vi "Measurement Logic.vi"() -> ()   [LabVIEW 2021, in "start-up.lvlib"]
uses:
  start-up.lvlib
  <vilib>/Plug-In SDKs/Measurements/Measure Call Context/Measure Call Context.lvclass
  Measurement Configuration.ctl
  Measurement Results.ctl
  Controls/LEDStartup_Data.ctl
  <instrlib>/niDCPower/nidcpower.llb/niDCPower Source Mode.ctl
  <instrlib>/niDCPower/nidcpower.llb/niDCPower Wait For Event - Event.ctl
  <instrlib>/niDCPower/nidcpower.llb/niDCPower Output Function.ctl
  <instrlib>/niDCPower/nidcpower.llb/niDCPower Sequence Attribute Type.ctl
  <instrlib>/niDCPower/nidcpower.llb/niDCPower Get Channel Name From String.vi
  <vilib>/Utility/error.llb/Error Cluster From Error Code.vi
  <instrlib>/niDCPower/nidcpower.llb/niDCPower Create Advanced Sequence Step With Channels.vi
  <instrlib>/niDCPower/nidcpower.llb/niDCPower Configure Digital Edge Source Trigger With Channels.vi
  <instrlib>/niDCPower/nidcpower.llb/niDCPower Configure Digital Edge Measure Trigger With Channels.vi
  <vilib>/ErrorRing/Error Ring.xnode
panel:
  out "measurement results":T1={"Status"="Empty", "Source voltages"=[0.0], "Load voltages"=[0.0], "Source current"=[0.0], "Load current"=[0.0]}
  in  "measurement configuration":T2={"Source resource name"="", "DUT setup time"=0.5, "Source delay"=0.5, "Aperture time"=0.001, "LED voltage (Vo)"=3.06, "LED current (Io)"=0.06, "Cumulative forward voltage (Vf)"=2.83, "Source sense"=1009, "Source current limit"=2.0, "Source maximum power"=20.0, "Source start voltage"=2.7, "Source stop voltage"=5.5, "Source voltage sweep points"=10, "Load resource name"="", "Load sense"=1009, "Load voltage level range"=60.0, "Load voltage limit"=6.0, "Max output resistance"="", "Load current limit range"="", "DUT current limit"=0.0} {"DUT current limit" format="%.3f"; "LED current (Io)" format="%.2f"; "LED voltage (Vo)" format="%.3f"; "Load sense" items=["Local"=1008, "Remote"=1009]; "Source stop voltage" format="%.3f"; "Source start voltage" format="%.3f"; "Source current limit" format="%.3f"; "Source sense" items=["Local"=1008, "Remote"=1009]; "Aperture time" format="%.2p"; "Source delay" format="%#_6p"; "DUT setup time" format="%#_6p"}
  out "measure call context out":refnum<class "Measure Call Context.lvclass">
  in  "measure call context in":refnum<class "Measure Call Context.lvclass">
  out "error out":errorcluster
  in  "error in":errorcluster
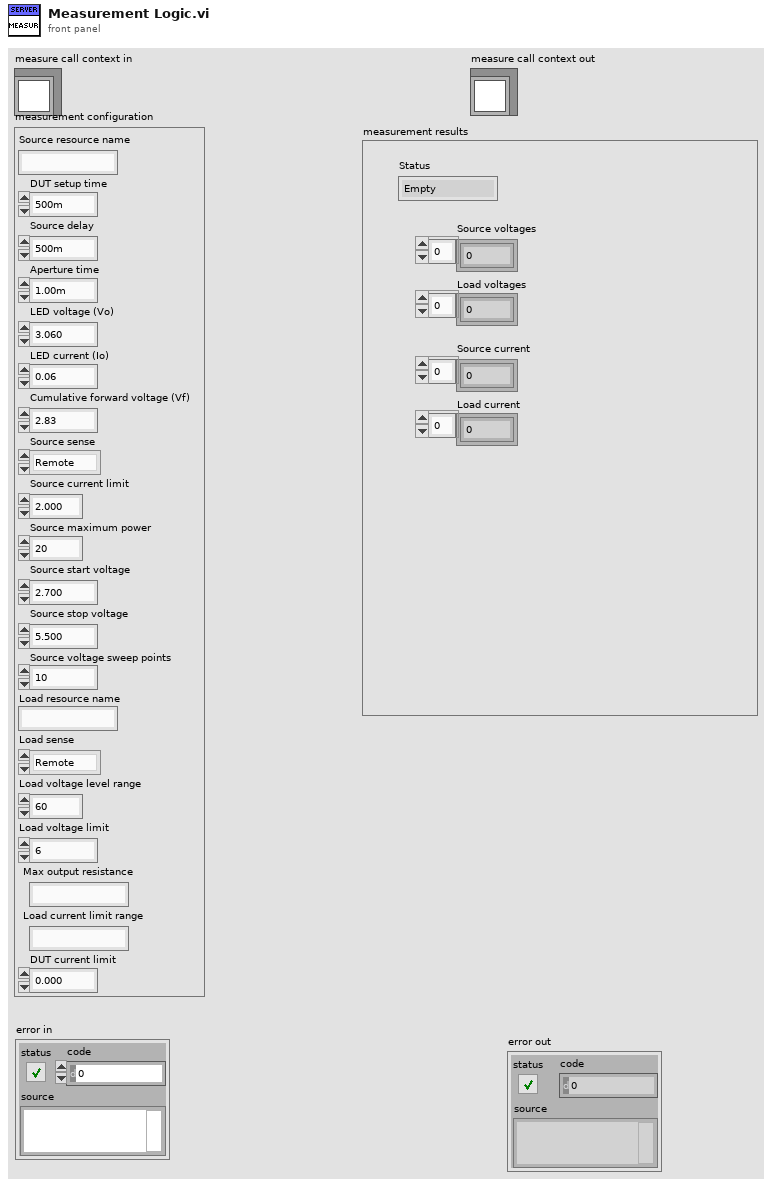
[diagram p1: front panel]
types:
  T1 = typedef "start-up.lvlib/Measurement Results.ctl" = cluster{"Status":string, "Source voltages":dbl[], "Load voltages":dbl[], "Source current":dbl[], "Load current":dbl[]}
  T2 = typedef "start-up.lvlib/Measurement Configuration.ctl" = cluster{"Source resource name":string, "DUT setup time":dbl, "Source delay":dbl, "Aperture time":dbl, "LED voltage (Vo)":dbl, "LED current (Io)":dbl, "Cumulative forward voltage (Vf)":dbl, "Source sense":i32, "Source current limit":dbl, "Source maximum power":dbl, "Source start voltage":dbl, "Source stop voltage":dbl, "Source voltage sweep points":i32, "Load resource name":string, "Load sense":i32, "Load voltage level range":dbl, "Load voltage limit":dbl, "Max output resistance":string, "Load current limit range":string, "DUT current limit":dbl}
  T3 = typedef "start-up.lvlib/LEDStartup_Data.ctl" = cluster{"Load channel name":string, "Load out":refnum<k15>, "Source out":refnum<k15>, "Source channel name":string, "Source sequence name":string, "Voltage values":dbl[], "Voltage values-CV":dbl[], "Voltage values-LED":dbl[], "Output Resistance-LED":dbl[], "Source terminal name":string, "Measure terminal name":string, "Load Voltage-out":dbl[], "Load Current - out":dbl[], "Source Voltage-out":dbl[], "Source Current - out":dbl[], "LED Mode Start?":bool, "LED Mode Completed?":bool, "CalculateRd":dbl, "Set LED Current Limit?":bool, "OutputVoltageOffset":dbl, "measurement results":T1}
  T4 = typedef "niDCPower Wait For Event - Event.ctl" = i32
  T5 = typedef "niDCPower Source Mode.ctl" = i32
  T6 = typedef "niDCPower Sequence Attribute Type.ctl" = i32
  T7 = typedef "niDCPower Output Function.ctl" = i32
  T8 = cluster{"Source Voltage":dbl[], "Source Current":dbl[], "Load Voltage":dbl[], "Load Current":dbl[]}
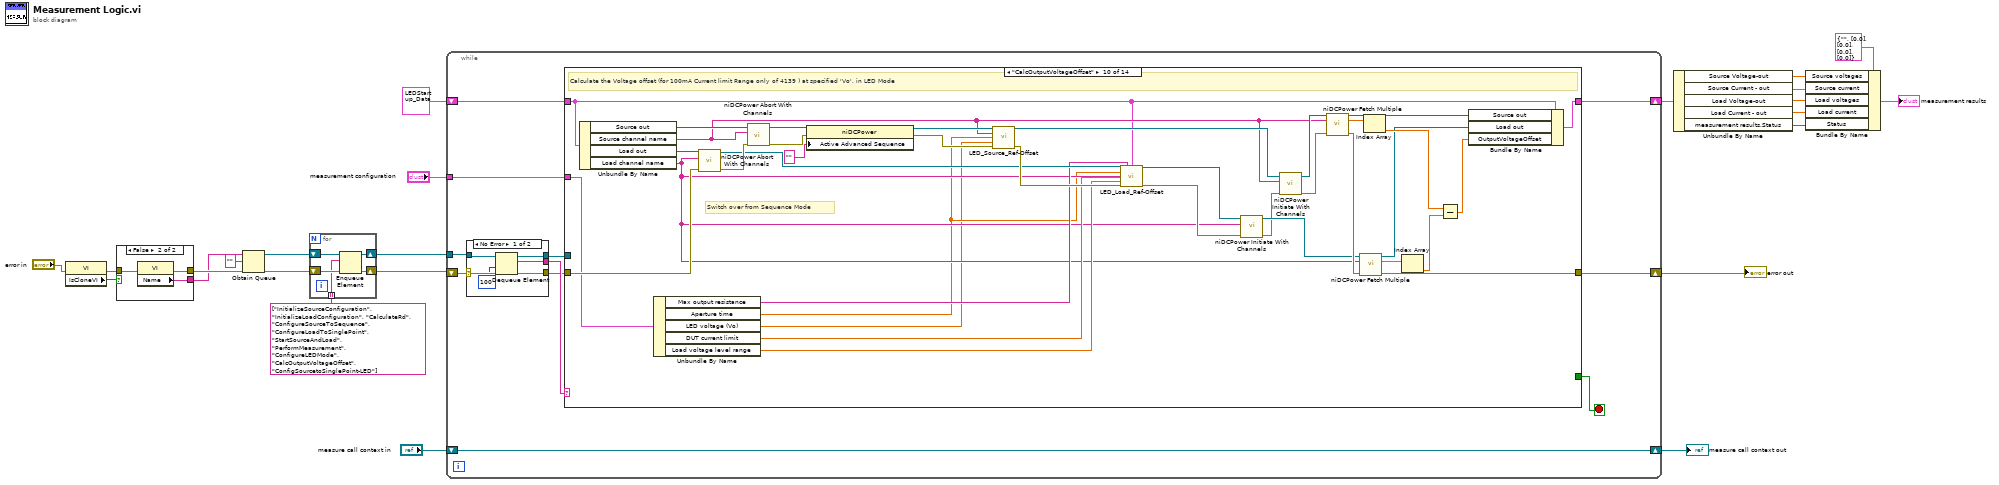
[diagram p0: block diagram]
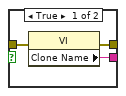
[diagram p2: hidden frame]
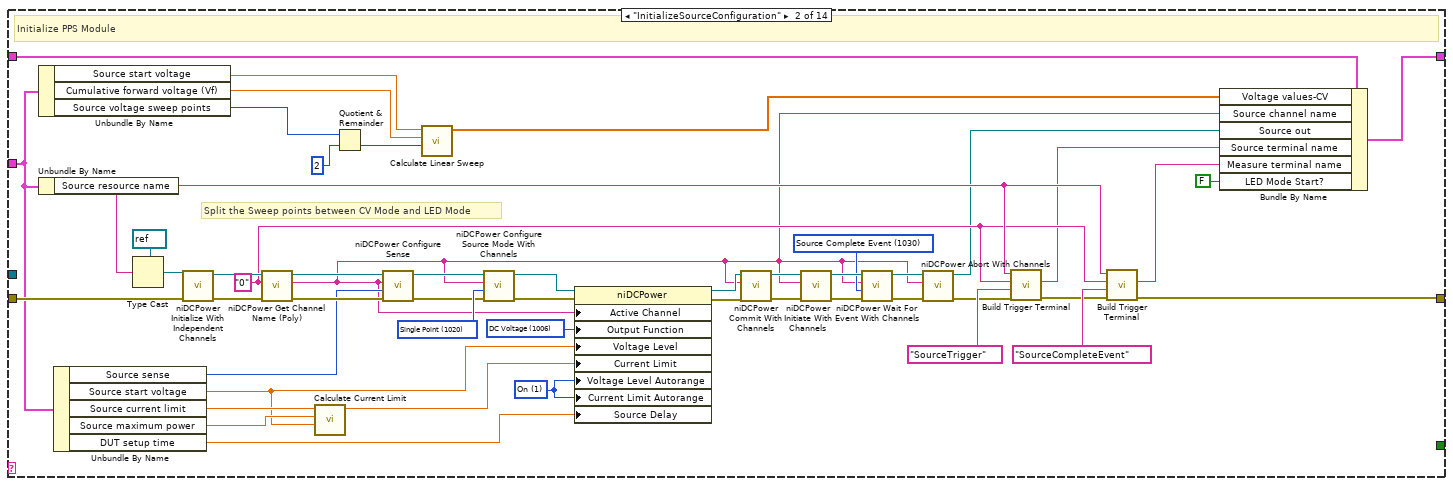
[diagram p4: hidden frame]
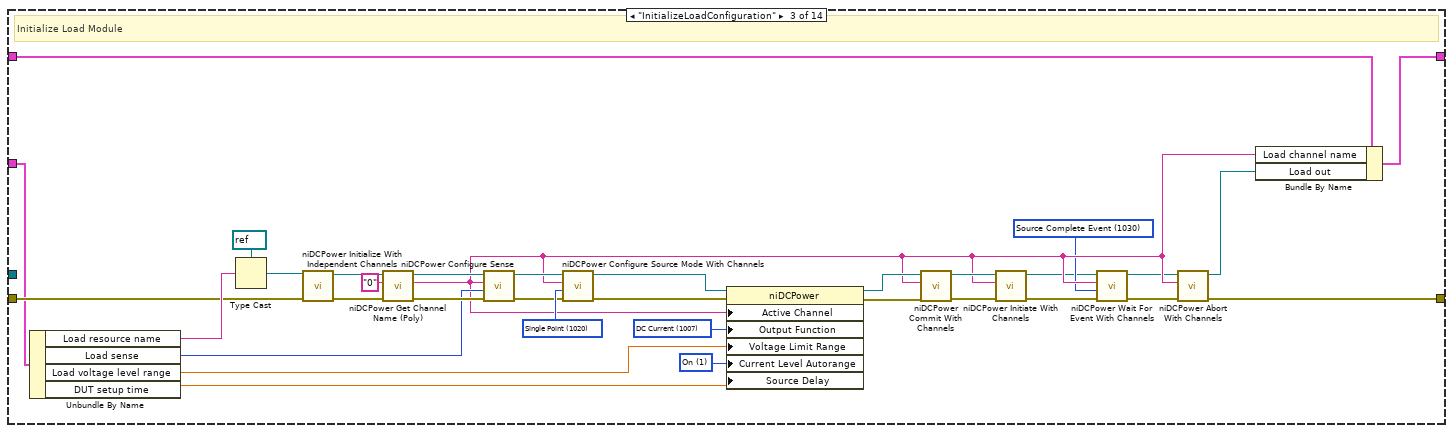
[diagram p5: hidden frame]
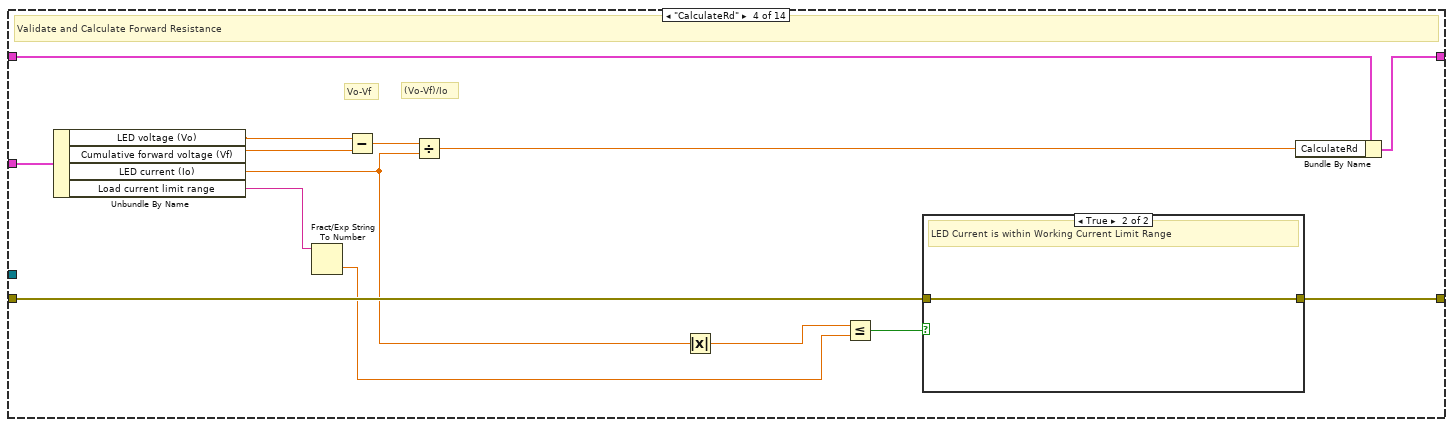
[diagram p6: hidden frame]
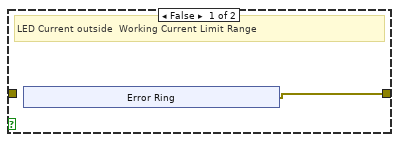
[diagram p7: hidden frame]
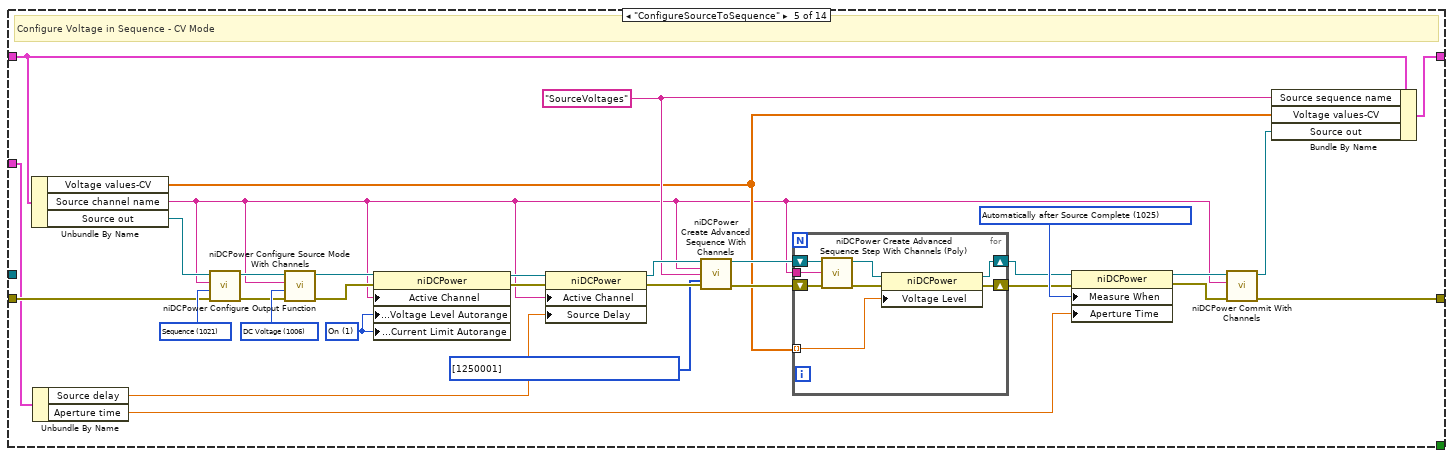
[diagram p8: hidden frame]
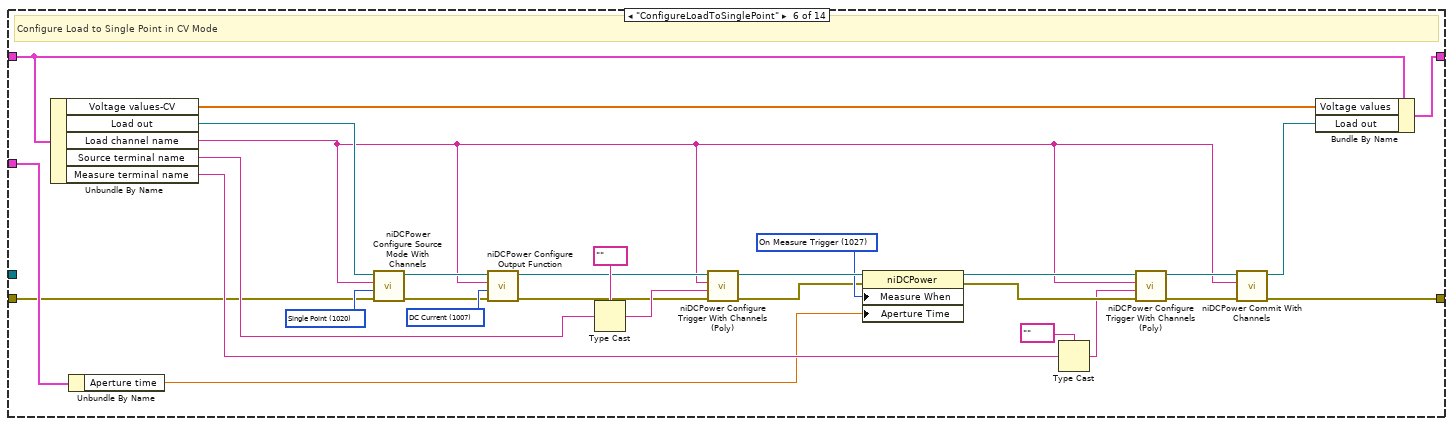
[diagram p9: hidden frame]
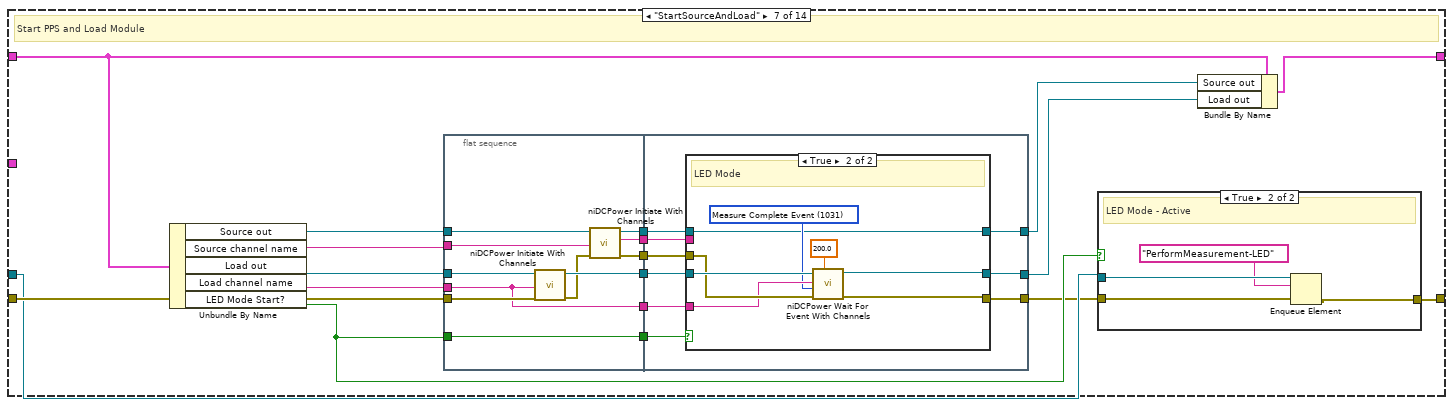
[diagram p10: hidden frame]
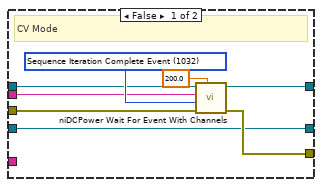
[diagram p12: hidden frame]
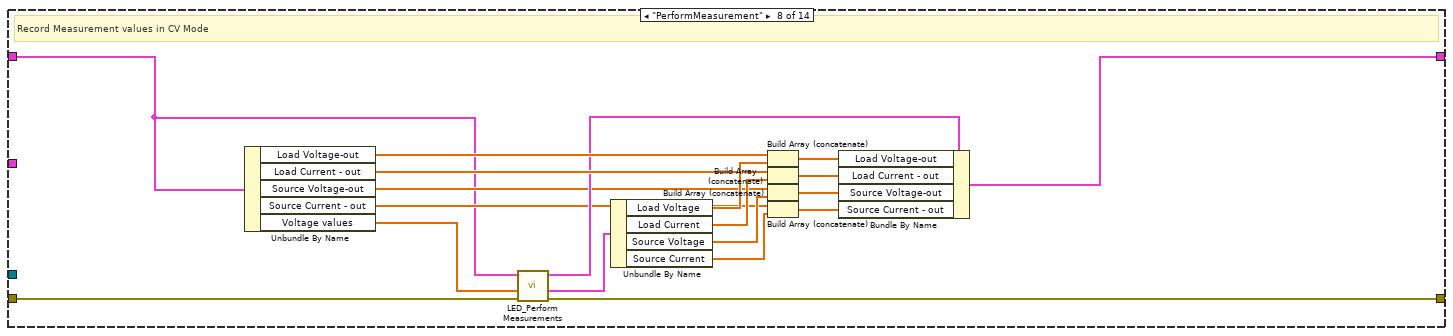
[diagram p13: hidden frame]
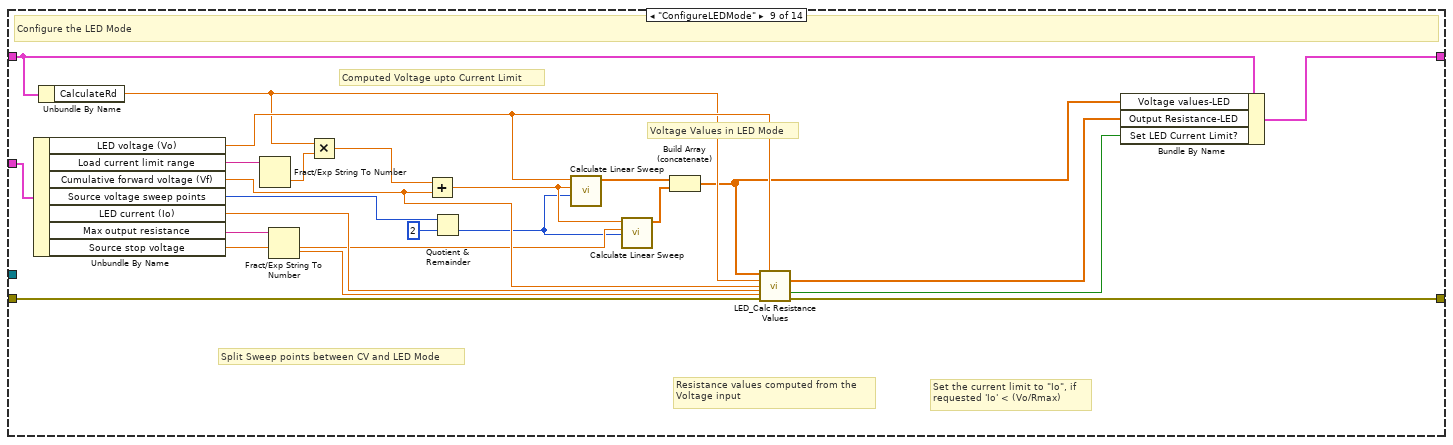
[diagram p14: hidden frame]
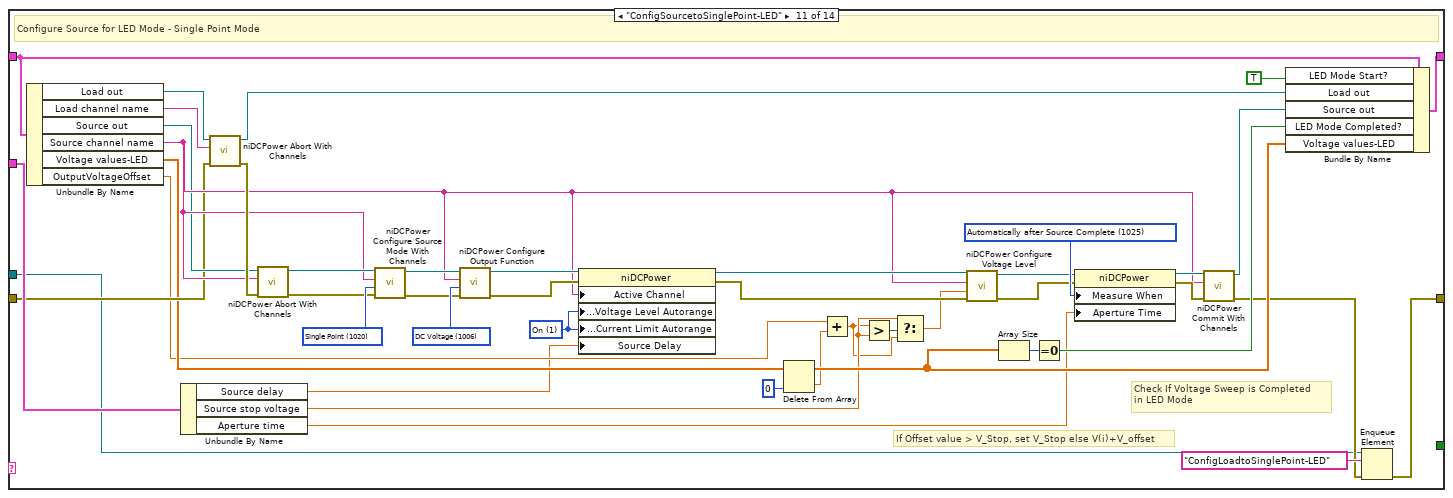
[diagram p15: hidden frame]
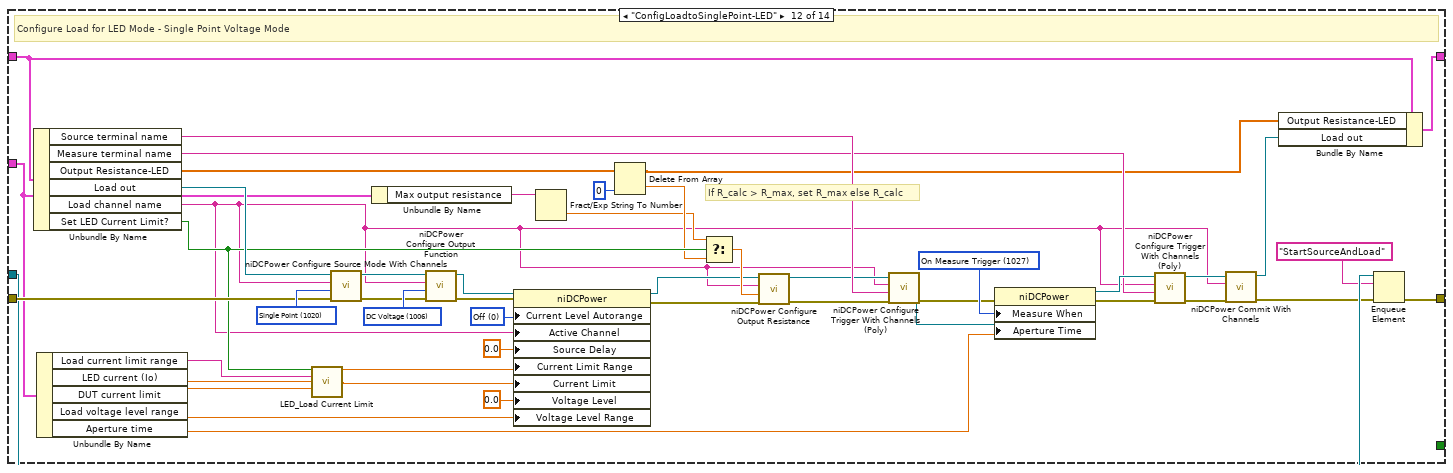
[diagram p16: hidden frame]
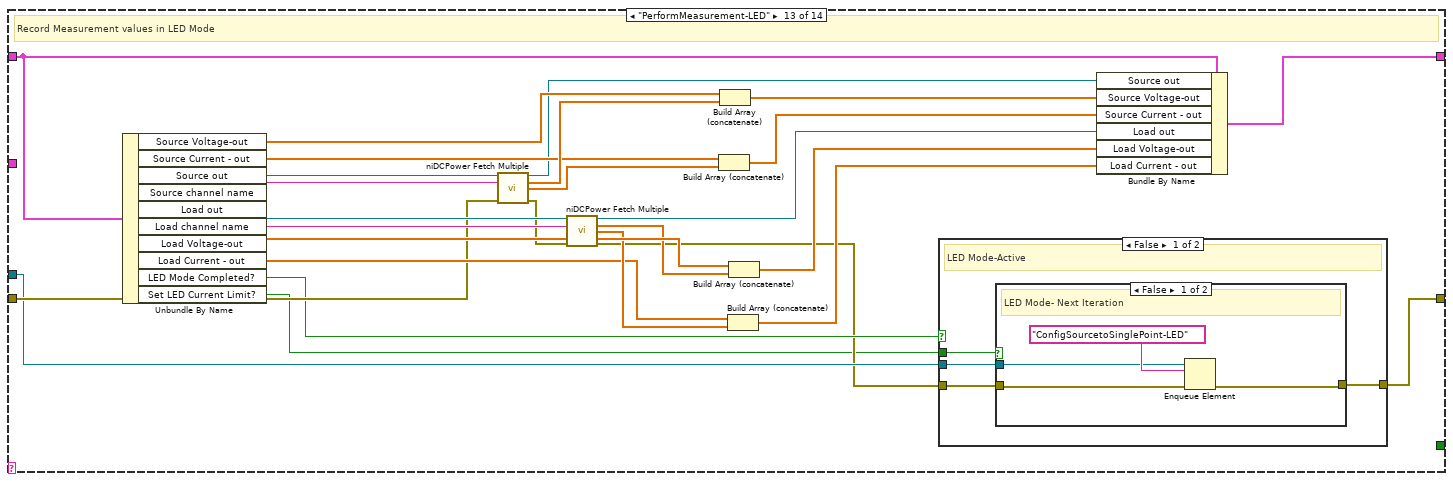
[diagram p17: hidden frame]
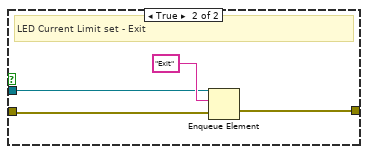
[diagram p18: hidden frame]
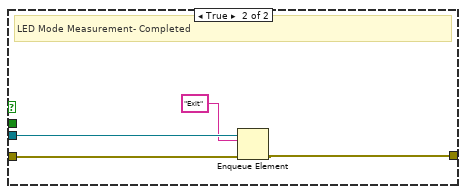
[diagram p19: hidden frame]
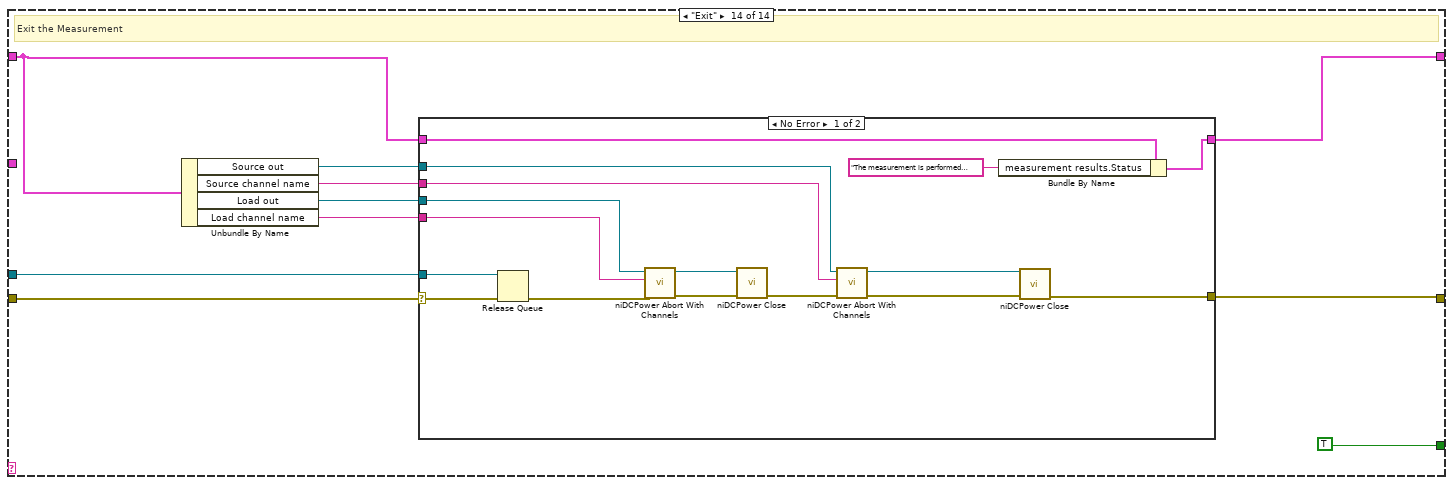
[diagram p20: hidden frame]
diagram:
  n1 = property class="VI"(error in="error in") -> (error out=w20:errorcluster, "IsCloneVI"=w21:bool)  [unwired: 1 in, 1 out]
  n2 = case shown="False" w21 {
    tunnel: [w27 w30] -> w14
    tunnel: [w26 w29] -> w13
    tunnel: w20 -> [w25 w28]
    frame True {
      n3 = property class="VI"(error in=w25) -> (error out=w27:errorcluster, "Clone Name"=w26:string)  [unwired: 1 in, 1 out]
    }
    frame False {
      n4 = property class="VI"(error in=w28) -> (error out=w30:errorcluster, "Name"=w29:string)  [unwired: 1 in, 1 out]
    }
  }
  n5 = Obtain Queue(name (unnamed)=w13, element data type="", error in (no error)=w14) -> (queue out=w17:refnum<queue>, error out=w18:errorcluster)  [unwired: 2 in, 1 out]
  n6 = for {
    shift-right: [w33] -> w11
    shift-left: w17 -> [w35]
    shift-right: [w32] -> w12
    shift-left: w18 -> [w34]
    tunnel: string[] ["InitializeSourceConfiguration", "InitializeLoadConfiguration", "CalculateRd", "ConfigureSourceToSequence", "ConfigureLoadToSinglePoint", "StartSourceAndLoad", "PerformMeasurement", "ConfigureLEDMode", "CalcOutputVoltageOffset", "ConfigSourcetoSinglePoint-LED"] ("Step sequence") -> [w31] mode=indexing
    n7 = Enqueue Element(queue=w35, element=w31, error in (no error)=w34) -> (queue out=w33:refnum<queue>, error out=w32:errorcluster)  [unwired: 1 in, 1 out]
  }
  n8 = while {
    shift-right: [w46] -> w23
    shift-left: "measure call context in" -> [w46]
    shift-right: [w39] -> w22
    shift-left: w12 -> [w45]
    tunnel: w11 -> [w44]
    tunnel: "measurement configuration" -> [w41]
    shift-right: [w38] -> w8
    shift-left: T3 {"Load channel name"="", "Load out"="", "Source out"="", "Source channel name"="", "Source sequence name"="", "Voltage values"=[], "Voltage values-CV"=[], "Voltage values-LED"=[], "Output Resistance-LED"=[], "Source terminal name"="", "Measure terminal name"="", "Load Voltage-out"=[], "Load Current - out"=[], "Source Voltage-out"=[], "Source Current - out"=[], "LED Mode Start?"=FALSE, "LED Mode Completed?"=FALSE, "CalculateRd"=0.0, "Set LED Current Limit?"=FALSE, "OutputVoltageOffset"=0.0, "measurement results"={"Status"="Empty", "Source voltages"=[0.0], "Load voltages"=[0.0], "Source current"=[0.0], "Load current"=[0.0]}} -> [w40]
    stop <- w36 stop-if-true
    n9 = case shown="No Error" w45 {
      selector: w45 -> [w546 w550]
      tunnel: w44 -> [w548 w549]
      tunnel: [w547 "Exit" ("t")] -> w43
      tunnel: [w545 w550] -> w42
      tunnel: [w543 w549] -> w37
      frame No Error {
        n10 = Dequeue Element(queue=w548, timeout in ms (-1)=100, error in (no error)=w546) -> (queue out=w543:refnum<queue>, element=w547:string, error out=w545:errorcluster)  [unwired: 1 out]
      }
      frame Error {
      }
    }
    n11 = case shown="\"CalcOutputVoltageOffset\"" w43 {
      tunnel: w42 -> [w47 w77 w113 w139 w170 w199 w232 w285 w313 w359 w381 w433 w460 w497]
      tunnel: w41 -> [_ w51 w109 w146 w159 w205 _ _ w323 w353 w392 w421 _ _]
      tunnel: w40 -> [w48 w57 w108 w143 w165 w202 w231 w286 w310 w326 w391 w438 w468 w501]
      tunnel: [w47 w60 w105 w135 w163 w194 w222 w281 w301 w330 w371 w416 w455 w502] -> w39
      tunnel: [w48 w59 w104 w142 w162 w200 w228 w283 w308 w339 w388 w436 w461 w500] -> w38
      tunnel: w37 -> [_ _ _ _ _ _ w224 _ _ _ w370 w418 w458 w498]
      tunnel: [_ _ _ _ _ _ _ _ _ _ _ _ _ TRUE] -> w36
      frame Default {
      }
      frame "InitializeSourceConfiguration" {
        w64 = "0" ("index")
        w71 = 1 items=["Off", "On"] ("Source:DC Voltage:Voltage Level Autorange")
        w83 = T4 1030 items=["Source Complete Event"=1030, "Measure Complete Event"=1031, "Sequence Iteration Complete Event"=1032, "Sequence Engine Done Event"=1033, "Pulse Complete Event"=1051, "Ready For Pulse Trigger Event"=1052] ("event")
        w94 = T5 1020 items=["Single Point"=1020, "Sequence"=1021] ("source mode")
        w89 = 1006 items=["DC Voltage"=1006, "DC Current"=1007, "Pulse Voltage"=1049, "Pulse Current"=1050] ("Source:Output Function")
        # "Split the Sweep points between CV Mode and LED Mode"
        # "Initialize PPS Module"
        n12 = Unbundle By Name(w51) -> ("Source start voltage"=w56:dbl, "Cumulative forward voltage (Vf)"=w55:dbl, "Source voltage sweep points"=w54:i32)
        n13 = Unbundle By Name(w51) -> ("Source resource name"=w65:string)
        n14 = Unbundle By Name(w51) -> ("Source sense"=w76:i32, "Source start voltage"=w72:dbl, "Source current limit"=w75:dbl, "Source maximum power"=w74:dbl, "DUT setup time"=w70:dbl)
        n15 = Type Cast(type=refnum<k15> refnum ("resource name"), x=w65) -> (*(type *) &x=w78:refnum<k15>)
        n16 = call <instrlib>:"niDCPower Initialize With Independent Channels.vi"("error in (no error)"=w77, "resource name"=w78) -> ("error out"=w81:errorcluster, "instrument handle out"=w84:refnum<k15>)  [unwired: 8 in]
        n17 = call-poly <instrlib>:"niDCPower Get Channel Name (Poly).vi"("error in (no error)"=w81, "index"=w64, "instrument handle"=w84) -> ("error out"=w80:errorcluster, "name"=w58:string, "instrument handle out"=w82:refnum<k15>)  [unwired: 6 in]
        n18 = call "Calculate Current Limit.vi"("Voltage value"=w72, "Maximum power"=w74, "Current limit in"=w75) -> ("Current limit out"=w73:dbl)  [unwired: 8 in]
        n19 = Quotient & Remainder(x=w54, y=2) -> (floor(x/y)=w53:i32)  [unwired: 1 out]
        n20 = call <instrlib>:"niDCPower Configure Sense.vi"("error in (no error)"=w80, "sense"=w76, "channel name"=w58, "instrument handle"=w82) -> ("error out"=w92:errorcluster, "instrument handle out"=w90:refnum<k15>)  [unwired: 6 in]
        n21 = call "Calculate Linear Sweep.vi"("Points"=w53, "Stop level"=w55, "Start level"=w56) -> ("Values"=w50:dbl[])  [unwired: 8 in]
        n22 = call <instrlib>:"niDCPower Configure Source Mode With Channels.vi"("error in (no error)"=w92, "source mode"=w94, "channel name"=w58, "instrument handle"=w90) -> ("error out"=w93:errorcluster, "instrument handle out"=w91:refnum<k15>)  [unwired: 6 in]
        n23 = property class="niDCPower"(reference=w91, error in=w93, "Active Channel"=w58, "Output Function"=w89, "Voltage Level"=w72, "Current Limit"=w73, "Voltage Level Autorange"=w71, "Current Limit Autorange"=w71, "Source Delay"=w70) -> (reference out=w95:refnum<k15>, error out=w96:errorcluster)
        n24 = call <instrlib>:"niDCPower Commit With Channels.vi"("error in (no error)"=w96, "channel name"=w58, "instrument handle"=w95) -> ("error out"=w98:errorcluster, "instrument handle out"=w97:refnum<k15>)  [unwired: 7 in]
        n25 = call <instrlib>:"niDCPower Initiate With Channels.vi"("error in (no error)"=w98, "channel name"=w58, "instrument handle"=w97) -> ("error out"=w85:errorcluster, "instrument handle out"=w86:refnum<k15>)  [unwired: 7 in]
        n26 = call <instrlib>:"niDCPower Wait For Event With Channels.vi"("error in (no error)"=w85, "event"=w83, "channel name"=w58, "instrument handle"=w86) -> ("error out"=w88:errorcluster, "instrument handle out"=w87:refnum<k15>)  [unwired: 6 in]
        n27 = call <instrlib>:"niDCPower Abort With Channels.vi"("error in (no error)"=w88, "channel name"=w58, "instrument handle"=w87) -> ("error out"=w67:errorcluster, "instrument handle out"=w63:refnum<k15>)  [unwired: 7 in]
        n28 = call "Build Trigger Terminal.vi"("error in (no error)"=w67, "Trigger/Event Name"="SourceTrigger", "Channel Name"=w64, "Resource Name"=w65) -> ("error out"=w66:errorcluster, "Terminal Name"=w62:string)  [unwired: 6 in]
        n29 = call "Build Trigger Terminal.vi"("error in (no error)"=w66, "Trigger/Event Name"="SourceCompleteEvent", "Channel Name"=w64, "Resource Name"=w65) -> ("error out"=w60:errorcluster, "Terminal Name"=w61:string)  [unwired: 6 in]
        n30 = Bundle By Name(cluster=w57, "Voltage values-CV"=w50, "Source channel name"=w58, "Source out"=w63, "Source terminal name"=w62, "Measure terminal name"=w61, "LED Mode Start?"=FALSE) -> (w59:T3)
      }
      frame "InitializeLoadConfiguration" {
        w101 = T4 1030 items=["Source Complete Event"=1030, "Measure Complete Event"=1031, "Sequence Iteration Complete Event"=1032, "Sequence Engine Done Event"=1033, "Pulse Complete Event"=1051, "Ready For Pulse Trigger Event"=1052] ("event")
        w128 = T5 1020 items=["Single Point"=1020, "Sequence"=1021] ("source mode")
        w121 = 1 items=["Off", "On"] ("Source:DC Current:Current Level Autorange")
        w122 = 1007 items=["DC Voltage"=1006, "DC Current"=1007, "Pulse Voltage"=1049, "Pulse Current"=1050] ("Source:Output Function")
        # "Initialize Load Module"
        n31 = Unbundle By Name(w109) -> ("Load resource name"=w115:string, "Load sense"=w112:i32, "Load voltage level range"=w111:dbl, "DUT setup time"=w110:dbl)
        n32 = Type Cast(type=refnum<k15> refnum ("resource name"), x=w115) -> (*(type *) &x=w114:refnum<k15>)
        n33 = call <instrlib>:"niDCPower Initialize With Independent Channels.vi"("error in (no error)"=w113, "resource name"=w114) -> ("error out"=w118:errorcluster, "instrument handle out"=w123:refnum<k15>)  [unwired: 8 in]
        n34 = call-poly <instrlib>:"niDCPower Get Channel Name (Poly).vi"("error in (no error)"=w118, "index"="0", "instrument handle"=w123) -> ("error out"=w117:errorcluster, "name"=w106:string, "instrument handle out"=w120:refnum<k15>)  [unwired: 6 in]
        n35 = call <instrlib>:"niDCPower Configure Sense.vi"("error in (no error)"=w117, "sense"=w112, "channel name"=w106, "instrument handle"=w120) -> ("error out"=w125:errorcluster, "instrument handle out"=w124:refnum<k15>)  [unwired: 6 in]
        n36 = call <instrlib>:"niDCPower Configure Source Mode With Channels.vi"("error in (no error)"=w125, "source mode"=w128, "channel name"=w106, "instrument handle"=w124) -> ("error out"=w127:errorcluster, "instrument handle out"=w126:refnum<k15>)  [unwired: 6 in]
        n37 = property class="niDCPower"(reference=w126, error in=w127, "Active Channel"=w106, "Output Function"=w122, "Voltage Limit Range"=w111, "Current Level Autorange"=w121, "Source Delay"=w110) -> (reference out=w129:refnum<k15>, error out=w130:errorcluster)
        n38 = call <instrlib>:"niDCPower Commit With Channels.vi"("error in (no error)"=w130, "channel name"=w106, "instrument handle"=w129) -> ("error out"=w131:errorcluster, "instrument handle out"=w132:refnum<k15>)  [unwired: 7 in]
        n39 = call <instrlib>:"niDCPower Initiate With Channels.vi"("error in (no error)"=w131, "channel name"=w106, "instrument handle"=w132) -> ("error out"=w99:errorcluster, "instrument handle out"=w100:refnum<k15>)  [unwired: 7 in]
        n40 = call <instrlib>:"niDCPower Wait For Event With Channels.vi"("error in (no error)"=w99, "event"=w101, "channel name"=w106, "instrument handle"=w100) -> ("error out"=w103:errorcluster, "instrument handle out"=w102:refnum<k15>)  [unwired: 6 in]
        n41 = call <instrlib>:"niDCPower Abort With Channels.vi"("error in (no error)"=w103, "channel name"=w106, "instrument handle"=w102) -> ("error out"=w105:errorcluster, "instrument handle out"=w107:refnum<k15>)  [unwired: 7 in]
        n42 = Bundle By Name(cluster=w108, "Load channel name"=w106, "Load out"=w107) -> (w104:T3)
      }
      frame "CalculateRd" {
        # "Vo-Vf"
        # "(Vo-Vf)/Io"
        # "Validate and Calculate Forward Resistance"
        n43 = Unbundle By Name(w146) -> ("LED voltage (Vo)"=w144:dbl, "Cumulative forward voltage (Vf)"=w138:dbl, "LED current (Io)"=w137:dbl, "Load current limit range"=w141:string)
        n44 = Fract/Exp String To Number(string=w141) -> (number=w136:dbl)  [unwired: 3 in, 1 out]
        n45 = Subtract(x=w144, y=w138) -> (x-y=w145:dbl)
        n46 = Divide(x=w145, y=w137) -> (x/y=w140:dbl)
        n47 = Absolute Value(x=w137) -> (abs(x)=w134:dbl)
        n48 = Less Or Equal?(x=w134, y=w136) -> (x <= y?=w133:bool)
        n49 = case shown="True" w133 {
          tunnel: [w147 w153] -> w135
          tunnel: w139 -> [_ w153]
          frame False {
            # "LED Current outside  Working Current Limit Range"
            n50 = xnode "Error Ring"() -> ("error out"=w147:errorcluster)
          }
          frame True {
            # "LED Current is within Working Current Limit Range"
          }
        }
        n51 = Bundle By Name(cluster=w143, "CalculateRd"=w140) -> (w142:T3)
      }
      frame "ConfigureSourceToSequence" {
        w166 = 1025 items=["Automatically after Source Complete"=1025, "On Demand"=1026, "On Measure Trigger"=1027] ("Measurement:Advanced:Measure When")
        w154 = 1 items=["Off", "On"] ("DC Voltage:Voltage Level Autorange")
        w167 = T6[] [1250001] items=["Source -> Output Function"=1150008, "Source -> Output Enabled"=1250006, "Source -> Output Resistance"=1150061, "Source -> Transient Response"=1150062, "Source -> Custom Transient Response -> Voltage Gain Bandwidth"=1150067, "Source -> Custom Transient Response -> Voltage Compensation Frequency"=1150068, "Source -> Custom Transient Response -> Voltage Pole-Zero Ratio"=1150069, "Source -> Custom Transient Response -> Current Gain Bandwidth"=1150070, "Source -> Custom Transient Response -> Current Compensation Frequency"=1150071, "Source -> Custom Transient Response -> Current Pole-Zero Ratio"=1150072, "Source -> DC Voltage -> Voltage Level"=1250001, "Source -> DC Voltage -> Voltage Level Range"=1150005, "Source -> DC Voltage -> Current Limit"=1250005, "Source -> DC Voltage -> Current Limit High"=1150187, "Source -> DC Voltage -> Current Limit Low"=1150188, "Source -> DC Voltage -> Current Limit Range"=1150004, "Source -> DC Current -> Current Level"=1150009, "Source -> DC Current -> Current Level Range"=1150011, "Source -> DC Current -> Voltage Limit"=1150010, "Source -> DC Current -> Voltage Limit High"=1150185, "Source -> DC Current -> Voltage Limit Low"=1150186, "Source -> DC Current -> Voltage Limit Range"=1150012, "Source -> Pulse Voltage -> Pulse Voltage Level"=1150080, "Source -> Pulse Voltage -> Pulse Bias Voltage Level"=1150082, "Source -> Pulse Voltage -> Pulse Voltage Level Range"=1150084, "Source -> Pulse Voltage -> Pulse Current Limit"=1150081, "Source -> Pulse Voltage -> Pulse Current Limit High"=1150193, "Source -> Pulse Voltage -> Pulse Current Limit Low"=1150194, "Source -> Pulse Voltage -> Pulse Bias Current Limit"=1150083, "Source -> Pulse Voltage -> Pulse Bias Current Limit High"=1150195, "Source -> Pulse Voltage -> Pulse Bias Current Limit Low"=1150196, "Source -> Pulse Voltage -> Pulse Current Limit Range"=1150085, "Source -> Pulse Current -> Pulse Current Level"=1150086, "Source -> Pulse Current -> Pulse Bias Current Level"=1150088, "Source -> Pulse Current -> Pulse Current Level Range"=1150090, "Source -> Pulse Current -> Pulse Voltage Limit"=1150087, "Source -> Pulse Current -> Pulse Voltage Limit High"=1150189, "Source -> Pulse Current -> Pulse Voltage Limit Low"=1150190, "Source -> Pulse Current -> Pulse Bias Voltage Limit"=1150089, "Source -> Pulse Current -> Pulse Bias Voltage Limit High"=1150191, "Source -> Pulse Current -> Pulse Bias Voltage Limit Low"=1150192, "Source -> Pulse Current -> Pulse Voltage Limit Range"=1150091, "Source -> Advanced -> Source Delay"=1150051, "Source -> Advanced -> Pulse Bias Delay"=1150092, "Source -> Advanced -> Pulse On Time"=1150093, "Source -> Advanced -> Pulse Off Time"=1150094, "Source -> Advanced -> OVP Enabled"=1250002, "Source -> Advanced -> OVP Limit"=1250003, "Source -> Advanced -> Compliance Limit Symmetry"=1150184, "Source -> Advanced -> Sequence Step Delta Time"=1150198, "Measurement -> Sense"=1150013, "Measurement -> Aperture Time"=1150058, "Measurement -> Measure Record Length"=1150063, "Measurement -> Advanced -> DC Noise Rejection"=1150066, "Measurement -> Autorange"=1150244, "Measurement -> Advanced -> Autorange Behavior"=1150245, "Measurement -> Advanced -> Autorange Aperture Time Mode"=1150246, "Measurement -> Advanced -> Autorange Minimum Aperture Time"=1150247, "Measurement -> Advanced -> Autorange Minimum Aperture Time Units"=1150248, "Measurement -> Advanced -> Autorange Minimum Current Range"=1150255, "Measurement -> Advanced -> Autorange Minimum Voltage Range"=1150256, "Measurement -> Advanced -> Autorange Threshold Mode"=1150257, "Measurement -> Advanced -> Autorange Maximum Delay After Range Change"=1150322, "LCR -> Instrument Mode"=1150208, "LCR -> LCR Stimulus Function"=1150209, "LCR -> LCR Frequency"=1150210, "LCR -> LCR Voltage Amplitude"=1150211, "LCR -> LCR Current Amplitude"=1150212, "LCR -> LCR DC Bias Source"=1150213, "LCR -> LCR DC Bias Voltage Level"=1150214, "LCR -> LCR DC Bias Current Level"=1150215, "LCR -> LCR Impedance Autorange"=1150216, "LCR -> LCR Impedance Range"=1150217, "LCR -> LCR Measurement Time"=1150218, "LCR -> LCR Custom Measurement Time"=1150258, "LCR -> LCR Source Delay Mode"=1150315, "LCR -> Compensation -> Open -> Enabled"=1150220, "LCR -> Compensation -> Open -> Conductance"=1150261, "LCR -> Compensation -> Open -> Susceptance"=1150262, "LCR -> Compensation -> Short -> Enabled"=1150221, "LCR -> Compensation -> Short -> Resistance"=1150263, "LCR -> Compensation -> Short -> Reactance"=1150264, "LCR -> Compensation -> Load -> Enabled"=1150222, "LCR -> Compensation -> Load -> Measured Resistance"=1150268, "LCR -> Compensation -> Load -> Measured Reactance"=1150269, "LCR -> Compensation -> Load -> Actual Resistance"=1150270, "LCR -> Compensation -> Load -> Actual Reactance"=1150271] ("advanced sequence properties")
        w164 = "SourceVoltages" ("sequence name")
        w176 = T7 1006 items=["DC Voltage"=1006, "DC Current"=1007, "Pulse Voltage"=1049, "Pulse Current"=1050] ("output function")
        w175 = T5 1021 items=["Single Point"=1020, "Sequence"=1021] ("source mode")
        # "Configure Voltage in Sequence - CV Mode"
        n52 = Unbundle By Name(w165) -> ("Voltage values-CV"=w158:dbl[], "Source channel name"=w155:string, "Source out"=w168:refnum<k15>)
        n53 = Unbundle By Name(w159) -> ("Source delay"=w169:dbl, "Aperture time"=w161:dbl)
        n54 = call <instrlib>:"niDCPower Configure Source Mode With Channels.vi"("error in (no error)"=w170, "source mode"=w175, "channel name"=w155, "instrument handle"=w168) -> ("error out"=w173:errorcluster, "instrument handle out"=w174:refnum<k15>)  [unwired: 6 in]
        n55 = call <instrlib>:"niDCPower Configure Output Function.vi"("error in (no error)"=w173, "output function"=w176, "channel name"=w155, "instrument handle"=w174) -> ("error out"=w182:errorcluster, "instrument handle out"=w181:refnum<k15>)  [unwired: 6 out]
        n56 = property class="niDCPower"(reference=w181, error in=w182, "Active Channel"=w155, "Source:DC Voltage:Voltage Level Autorange"=w154, "Source:DC Voltage:Current Limit Autorange"=w154) -> (reference out=w179:refnum<k15>, error out=w180:errorcluster)
        n57 = property class="niDCPower"(reference=w179, error in=w180, "Active Channel"=w155, "Source Delay"=w169) -> (reference out=w183:refnum<k15>, error out=w184:errorcluster)
        n58 = call <instrlib>:"niDCPower Create Advanced Sequence With Channels.vi"("instrument handle"=w183, "channel name"=w155, "sequence name"=w164, "advanced sequence properties"=w167, "error in (no error)"=w184) -> ("instrument handle out"=w177:refnum<k15>, "error out"=w178:errorcluster)  [unwired: 9 in]
        n59 = for {
          shift-right: [w189] -> w156
          shift-left: w178 -> [w192]
          shift-right: [w188] -> w157
          shift-left: w177 -> [w187]
          tunnel: w158 -> [w185] mode=indexing
          tunnel: w155 -> [w186]
          n60 = call-poly <instrlib>:"niDCPower Create Advanced Sequence Step With Channels (Poly).vi"("error in (no error)"=w192, "channel name"=w186, "instrument handle"=w187) -> ("error out"=w190:errorcluster, "instrument handle out"=w191:refnum<k15>)  [unwired: 7 in]
          n61 = property class="niDCPower"(reference=w191, error in=w190, "Voltage Level"=w185) -> (reference out=w188:refnum<k15>, error out=w189:errorcluster)
        }
        n62 = property class="niDCPower"(reference=w157, error in=w156, "Measure When"=w166, "Aperture Time"=w161) -> (reference out=w171:refnum<k15>, error out=w172:errorcluster)
        n63 = call <instrlib>:"niDCPower Commit With Channels.vi"("error in (no error)"=w172, "channel name"=w155, "instrument handle"=w171) -> ("error out"=w163:errorcluster, "instrument handle out"=w160:refnum<k15>)  [unwired: 7 in]
        n64 = Bundle By Name(cluster=w165, "Source sequence name"=w164, "Voltage values-CV"=w158, "Source out"=w160) -> (w162:T3)
      }
      frame "ConfigureLoadToSinglePoint" {
        w218 = T7 1007 items=["DC Voltage"=1006, "DC Current"=1007, "Pulse Voltage"=1049, "Pulse Current"=1050] ("output function")
        w217 = 1027 items=["Automatically after Source Complete"=1025, "On Demand"=1026, "On Measure Trigger"=1027] ("Measurement:Advanced:Measure When")
        w216 = T5 1020 items=["Single Point"=1020, "Sequence"=1021] ("source mode")
        # "Configure Load to Single Point in CV Mode"
        n65 = Unbundle By Name(w202) -> ("Voltage values-CV"=w201:dbl[], "Load out"=w198:refnum<k15>, "Load channel name"=w195:string, "Source terminal name"=w203:string, "Measure terminal name"=w206:string)
        n66 = Unbundle By Name(w205) -> ("Aperture time"=w204:dbl)
        n67 = call <instrlib>:"niDCPower Configure Source Mode With Channels.vi"("error in (no error)"=w199, "source mode"=w216, "channel name"=w195, "instrument handle"=w198) -> ("error out"=w214:errorcluster, "instrument handle out"=w215:refnum<k15>)  [unwired: 6 in]
        n68 = call <instrlib>:"niDCPower Configure Output Function.vi"("error in (no error)"=w214, "output function"=w218, "channel name"=w195, "instrument handle"=w215) -> ("error out"=w197:errorcluster, "instrument handle out"=w196:refnum<k15>)  [unwired: 6 in]
        n69 = Type Cast(type=tag "" ("input terminal"), x=w203) -> (*(type *) &x=w209:tag)
        n70 = call-poly <instrlib>:"niDCPower Configure Trigger With Channels (Poly).vi"("error in (no error)"=w197, "input terminal"=w209, "channel name"=w195, "instrument handle"=w196) -> ("error out"=w211:errorcluster, "instrument handle out"=w221:refnum<k15>)  [unwired: 6 in]
        n71 = property class="niDCPower"(reference=w221, error in=w211, "Measure When"=w217, "Aperture Time"=w204) -> (reference out=w213:refnum<k15>, error out=w212:errorcluster)
        n72 = Type Cast(type=tag "" ("input terminal"), x=w206) -> (*(type *) &x=w207:tag)
        n73 = call-poly <instrlib>:"niDCPower Configure Trigger With Channels (Poly).vi"("error in (no error)"=w212, "input terminal"=w207, "channel name"=w195, "instrument handle"=w213) -> ("error out"=w219:errorcluster, "instrument handle out"=w220:refnum<k15>)  [unwired: 6 in]
        n74 = call <instrlib>:"niDCPower Commit With Channels.vi"("error in (no error)"=w219, "channel name"=w195, "instrument handle"=w220) -> ("error out"=w194:errorcluster, "instrument handle out"=w193:refnum<k15>)  [unwired: 7 in]
        n75 = Bundle By Name(cluster=w202, "Voltage values"=w201, "Load out"=w193) -> (w200:T3)
      }
      frame "StartSourceAndLoad" {
        # "Start PPS and Load Module"
        n76 = Unbundle By Name(w231) -> ("Source out"=w236:refnum<k15>, "Source channel name"=w235:string, "Load out"=w234:refnum<k15>, "Load channel name"=w233:string, "LED Mode Start?"=w225:bool)
        n77 = flat-sequence {
          tunnel: [w255] -> w240
          tunnel: [w254] -> w239
          tunnel: [w253] -> w238
          tunnel: w232 -> [w252]
          tunnel: w234 -> [w251]
          tunnel: w236 -> [w250]
          tunnel: w235 -> [w249]
          tunnel: w233 -> [w248]
          tunnel: [w249] -> w237
          tunnel: [w247] -> w227
          tunnel: w225 -> [w247]
          tunnel: [w248] -> w226
          tunnel: w240 -> [w264]
          tunnel: w239 -> [w263]
          tunnel: w238 -> [w258]
          tunnel: [w261] -> w230
          tunnel: [w262] -> w223
          tunnel: [w257] -> w229
          tunnel: w237 -> [w260]
          tunnel: w227 -> [w259]
          tunnel: w226 -> [w256]
          frame #0 {
            n78 = call <instrlib>:"niDCPower Initiate With Channels.vi"("error in (no error)"=w252, "channel name"=w248, "instrument handle"=w251) -> ("error out"=w246:errorcluster, "instrument handle out"=w253:refnum<k15>)  [unwired: 7 in]
            n79 = call <instrlib>:"niDCPower Initiate With Channels.vi"("error in (no error)"=w246, "channel name"=w249, "instrument handle"=w250) -> ("error out"=w254:errorcluster, "instrument handle out"=w255:refnum<k15>)  [unwired: 7 in]
          }
          frame #1 {
            n80 = case shown="True" w259 {
              tunnel: w264 -> [w271 w274]
              tunnel: w263 -> [w270 w279]
              tunnel: [w269 w273] -> w262
              tunnel: [w268 w274] -> w261
              tunnel: w260 -> [w267 _]
              tunnel: [w265 w275] -> w257
              tunnel: w258 -> [w265 w280]
              tunnel: w256 -> [_ w278]
              frame False {
                w272 = T4 1032 items=["Source Complete Event"=1030, "Measure Complete Event"=1031, "Sequence Iteration Complete Event"=1032, "Sequence Engine Done Event"=1033] ("event")
                # "CV Mode"
                n81 = call <instrlib>:"niDCPower Wait For Event With Channels.vi"("timeout (10.0)"=200.0, "error in (no error)"=w270, "event"=w272, "channel name"=w267, "instrument handle"=w271) -> ("error out"=w269:errorcluster, "instrument handle out"=w268:refnum<k15>)  [unwired: 5 in]
              }
              frame True {
                w277 = T4 1031 items=["Source Complete Event"=1030, "Measure Complete Event"=1031, "Sequence Iteration Complete Event"=1032, "Sequence Engine Done Event"=1033, "Pulse Complete Event"=1051, "Ready For Pulse Trigger Event"=1052] ("event")
                # "LED Mode"
                n82 = call <instrlib>:"niDCPower Wait For Event With Channels.vi"("timeout (10.0)"=200.0, "error in (no error)"=w279, "event"=w277, "channel name"=w278, "instrument handle"=w280) -> ("error out"=w273:errorcluster, "instrument handle out"=w275:refnum<k15>)  [unwired: 5 in]
              }
            }
          }
        }
        n83 = case shown="True" w225 {
          tunnel: w224 -> [_ w245]
          tunnel: w223 -> [w241 w244]
          tunnel: [w241 w243] -> w222
          frame False {
            # "LED Mode- Not Started"
          }
          frame True {
            # "LED Mode - Active"
            n84 = Enqueue Element(queue=w245, element="PerformMeasurement-LED", error in (no error)=w244) -> (error out=w243:errorcluster)  [unwired: 1 in, 2 out]
          }
        }
        n85 = Bundle By Name(cluster=w231, "Source out"=w230, "Load out"=w229) -> (w228:T3)
      }
      frame "PerformMeasurement" {
        # "Record Measurement values in CV Mode"
        n86 = Unbundle By Name(w286) -> ("Load Voltage-out"=w298:dbl[], "Load Current - out"=w295:dbl[], "Source Voltage-out"=w292:dbl[], "Source Current - out"=w288:dbl[], "Voltage values"=w282:dbl[])
        n87 = call "LED_Perform Measurements.vi"("error in"=w285, "Voltage Values"=w282, "Measurement Config_In"=w286) -> ("error Out"=w281:errorcluster, "Measurement Data"=w284:T8, "Measurement Config_Out"=w293:T3)  [unwired: 6 in]
        n88 = Unbundle By Name(w284) -> ("Load Voltage"=w299:dbl[], "Load Current"=w296:dbl[], "Source Voltage"=w290:dbl[], "Source Current"=w289:dbl[])
        n89 = Build Array (concatenate)(w298, w299) -> (w297:dbl[])
        n90 = Build Array (concatenate)(w295, w296) -> (w294:dbl[])
        n91 = Build Array (concatenate)(w292, w290) -> (w291:dbl[])
        n92 = Build Array (concatenate)(w288, w289) -> (w287:dbl[])
        n93 = Bundle By Name(cluster=w293, "Load Voltage-out"=w297, "Load Current - out"=w294, "Source Voltage-out"=w291, "Source Current - out"=w287) -> (w283:T3)
      }
      frame "ConfigureLEDMode" {
        # "Computed Voltage upto Current Limit"
        # "Set the current limit to \"Io\", if \nrequested 'Io' < (Vo/Rmax)"
        # "Resistance values computed from the\nVoltage input"
        # "Split Sweep points between CV and LED Mode"
        # "Voltage Values in LED Mode"
        # "Configure the LED Mode"
        n94 = Unbundle By Name(w323) -> ("LED voltage (Vo)"=w316:dbl, "Load current limit range"=w322:string, "Cumulative forward voltage (Vf)"=w311:dbl, "Source voltage sweep points"=w318:i32, "LED current (Io)"=w317:dbl, "Max output resistance"=w315:string, "Source stop voltage"=w306:dbl)
        n95 = Unbundle By Name(w310) -> ("CalculateRd"=w312:dbl)
        n96 = Fract/Exp String To Number(string=w322) -> (number=w321:dbl)  [unwired: 3 in, 1 out]
        n97 = Fract/Exp String To Number(string=w315) -> (number=w314:dbl)  [unwired: 3 in, 1 out]
        n98 = Multiply(x=w312, y=w321) -> (x*y=w320:dbl)
        n99 = Add(x=w320, y=w311) -> (x+y=w307:dbl)
        n100 = Quotient & Remainder(x=w318, y=2) -> (floor(x/y)=w305:i32)  [unwired: 1 out]
        n101 = call "Calculate Linear Sweep.vi"("Points"=w305, "Stop level"=w307, "Start level"=w316) -> ("Values"=w304:dbl[])  [unwired: 8 in]
        n102 = call "Calculate Linear Sweep.vi"("Points"=w305, "Stop level"=w306, "Start level"=w307) -> ("Values"=w303:dbl[])  [unwired: 8 in]
        n103 = Build Array (concatenate)(w304, w303) -> (w302:dbl[])
        n104 = call "LED_Calc Resistance Values.vi"("LED-Voltage Values"=w302, "LED Output Voltage(Vo)"=w316, "LED Forward Resistance(Rd)"=w312, "LED Forward Voltage (Vf)"=w311, "LED Current (Io)"=w317, "error in"=w313, "Max Resistance range"=w314) -> ("Resistance Values"=w309:dbl[], "Set LED Current Limit?"=w300:bool, "error out"=w301:errorcluster)  [unwired: 6 in]
        n105 = Bundle By Name(cluster=w310, "Voltage values-LED"=w302, "Output Resistance-LED"=w309, "Set LED Current Limit?"=w300) -> (w308:T3)
      }
      frame "CalcOutputVoltageOffset" {
        # "Switch over from Sequence Mode"
        # "Calculate the Voltage offset (for 100mA Current limit Range only of 4139 ) at specified 'Vo', in LED Mode"
        n106 = Unbundle By Name(w326) -> ("Source out"=w358:refnum<k15>, "Source channel name"=w331:string, "Load out"=w360:refnum<k15>, "Load channel name"=w327:string)
        n107 = Unbundle By Name(w353) -> ("Max output resistance"=w349:string, "Aperture time"=w325:dbl, "LED voltage (Vo)"=w324:dbl, "DUT current limit"=w328:dbl, "Load voltage level range"=w348:dbl)
        n108 = call <instrlib>:"niDCPower Abort With Channels.vi"("error in (no error)"=w359, "channel name"=w327, "instrument handle"=w360) -> ("error out"=w357:errorcluster, "instrument handle out"=w350:refnum<k15>)  [unwired: 7 in]
        n109 = call <instrlib>:"niDCPower Abort With Channels.vi"("error in (no error)"=w357, "channel name"=w331, "instrument handle"=w358) -> ("error out"=w354:errorcluster, "instrument handle out"=w355:refnum<k15>)  [unwired: 7 in]
        n110 = property class="niDCPower"(reference=w355, error in=w354, "Active Advanced Sequence"="" ("Source:Advanced:Active Advanced Sequence")) -> (reference out=w338:refnum<k15>, error out=w352:errorcluster)
        n111 = call "LED_Source_Ref-Offset.vi"("Source Resource In"=w338, "Source channel name"=w331, "Aperture time"=w325, "LED Voltage (Vo)"=w324, "error in"=w352) -> ("Source Resource Out"=w334:refnum<k15>, "error out"=w351:errorcluster)  [unwired: 9 in]
        n112 = call "LED_Load_Ref-Offset.vi"("Load Resource in"=w350, "Max Output Resistance"=w349, "Cluster"=w326, "Aperture time"=w325, "Load channel name"=w327, "DUT Current Limit"=w328, "error in"=w351, "Load voltage limit range"=w348) -> ("Load Resource Out"=w336:refnum<k15>, "error out"=w337:errorcluster)  [unwired: 6 in]
        n113 = call <instrlib>:"niDCPower Initiate With Channels.vi"("error in (no error)"=w337, "channel name"=w327, "instrument handle"=w336) -> ("error out"=w332:errorcluster, "instrument handle out"=w335:refnum<k15>)  [unwired: 7 in]
        n114 = call <instrlib>:"niDCPower Initiate With Channels.vi"("error in (no error)"=w332, "channel name"=w331, "instrument handle"=w334) -> ("error out"=w329:errorcluster, "instrument handle out"=w333:refnum<k15>)  [unwired: 7 in]
        n115 = call <instrlib>:"niDCPower Fetch Multiple.vi"("instrument handle"=w333, "channel name"=w331, "error in (no error)"=w329) -> ("instrument handle out"=w342:refnum<k15>, "voltage measurements"=w346:dbl[], "error out"=w347:errorcluster)  [unwired: 7 in, 3 out]
        n116 = call <instrlib>:"niDCPower Fetch Multiple.vi"("instrument handle"=w335, "channel name"=w327, "error in (no error)"=w347) -> ("instrument handle out"=w341:refnum<k15>, "voltage measurements"=w345:dbl[], "error out"=w330:errorcluster)  [unwired: 7 in, 3 out]
        n117 = Index Array(array=w346) -> (element=w344:dbl)  [unwired: 1 in]
        n118 = Index Array(array=w345) -> (element=w343:dbl)  [unwired: 1 in]
        n119 = Subtract(x=w344, y=w343) -> (x-y=w340:dbl)
        n120 = Bundle By Name(cluster=w326, "Source out"=w342, "Load out"=w341, "OutputVoltageOffset"=w340) -> (w339:T3)
      }
      frame "ConfigSourcetoSinglePoint-LED" {
        w398 = 1025 items=["Automatically after Source Complete"=1025, "On Demand"=1026, "On Measure Trigger"=1027] ("Measurement:Advanced:Measure When")
        w394 = 1 items=["Off", "On"] ("DC Voltage:Voltage Level Autorange")
        w401 = T7 1006 items=["DC Voltage"=1006, "DC Current"=1007, "Pulse Voltage"=1049, "Pulse Current"=1050] ("output function")
        w387 = T5 1020 items=["Single Point"=1020, "Sequence"=1021] ("source mode")
        # "Check If Voltage Sweep is Completed\nin LED Mode"
        # "If Offset value > V_Stop, set V_Stop else V(i)+V_offset"
        # "Configure Source for LED Mode - Single Point Mode"
        n121 = Unbundle By Name(w391) -> ("Load out"=w389:refnum<k15>, "Load channel name"=w393:string, "Source out"=w382:refnum<k15>, "Source channel name"=w383:string, "Voltage values-LED"=w380:dbl[], "OutputVoltageOffset"=w367:dbl)
        n122 = Unbundle By Name(w392) -> ("Source delay"=w361:dbl, "Source stop voltage"=w364:dbl, "Aperture time"=w366:dbl)
        n123 = call <instrlib>:"niDCPower Abort With Channels.vi"("error in (no error)"=w381, "channel name"=w393, "instrument handle"=w389) -> ("error out"=w395:errorcluster, "instrument handle out"=w369:refnum<k15>)  [unwired: 7 in]
        n124 = call <instrlib>:"niDCPower Abort With Channels.vi"("error in (no error)"=w395, "channel name"=w383, "instrument handle"=w382) -> ("error out"=w385:errorcluster, "instrument handle out"=w386:refnum<k15>)  [unwired: 7 in]
        n125 = call <instrlib>:"niDCPower Configure Source Mode With Channels.vi"("error in (no error)"=w385, "source mode"=w387, "channel name"=w383, "instrument handle"=w386) -> ("error out"=w399:errorcluster, "instrument handle out"=w400:refnum<k15>)  [unwired: 6 in]
        n126 = call <instrlib>:"niDCPower Configure Output Function.vi"("error in (no error)"=w399, "output function"=w401, "channel name"=w383, "instrument handle"=w400) -> ("error out"=w405:errorcluster, "instrument handle out"=w404:refnum<k15>)  [unwired: 6 out]
        n127 = property class="niDCPower"(reference=w404, error in=w405, "Active Channel"=w383, "Source:DC Voltage:Voltage Level Autorange"=w394, "Source:DC Voltage:Current Limit Autorange"=w394, "Source Delay"=w361) -> (reference out=w402:refnum<k15>, error out=w403:errorcluster)
        n128 = Delete From Array(array=w380, index=0) -> (deleted portion=w368:dbl, array with subset deleted=w375:dbl[])  [unwired: 1 in]
        n129 = Add(x=w367, y=w368) -> (x+y=w363:dbl)
        n130 = Greater?(x=w363, y=w364) -> (0:w365:bool)
        n131 = Select(t=w364, s=w365, f=w363) -> (s? t:f=w362:dbl)
        n132 = call <instrlib>:"niDCPower Configure Voltage Level.vi"("error in (no error)"=w403, "voltage level"=w362, "channel name"=w383, "instrument handle"=w402) -> ("error out"=w377:errorcluster, "instrument handle out"=w384:refnum<k15>)  [unwired: 6 in]
        n133 = Array Size(array=w375) -> (size(s)=w378:i32)
        n134 = Equal To 0?(x=w378) -> (x = 0?=w376:bool)
        n135 = property class="niDCPower"(reference=w384, error in=w377, "Measure When"=w398, "Aperture Time"=w366) -> (reference out=w396:refnum<k15>, error out=w397:errorcluster)
        n136 = call <instrlib>:"niDCPower Commit With Channels.vi"("error in (no error)"=w397, "channel name"=w383, "instrument handle"=w396) -> ("error out"=w372:errorcluster, "instrument handle out"=w390:refnum<k15>)  [unwired: 7 in]
        n137 = Bundle By Name(cluster=w391, "LED Mode Start?"=TRUE, "Load out"=w369, "Source out"=w390, "LED Mode Completed?"=w376, "Voltage values-LED"=w375) -> (w388:T3)
        n138 = Enqueue Element(queue=w370, element="ConfigLoadtoSinglePoint-LED", error in (no error)=w372) -> (error out=w371:errorcluster)  [unwired: 1 in, 2 out]
      }
      frame "ConfigLoadtoSinglePoint-LED" {
        w440 = 0 items=["Off", "On"] ("Source:DC Current:Current Level Autorange")
        w450 = T7 1006 items=["DC Voltage"=1006, "DC Current"=1007, "Pulse Voltage"=1049, "Pulse Current"=1050] ("output function")
        w449 = 1027 items=["Automatically after Source Complete"=1025, "On Demand"=1026, "On Measure Trigger"=1027] ("Measurement:Advanced:Measure When")
        w448 = T5 1020 items=["Single Point"=1020, "Sequence"=1021] ("source mode")
        # "If R_calc > R_max, set R_max else R_calc"
        # "Configure Load for LED Mode - Single Point Voltage Mode"
        n139 = Unbundle By Name(w438) -> ("Source terminal name"=w435:string, "Measure terminal name"=w434:string, "Output Resistance-LED"=w427:dbl[], "Load out"=w428:refnum<k15>, "Load channel name"=w408:string, "Set LED Current Limit?"=w424:bool)
        n140 = Unbundle By Name(w421) -> ("Load current limit range"=w431:string, "LED current (Io)"=w429:dbl, "DUT current limit"=w412:dbl, "Load voltage level range"=w414:dbl, "Aperture time"=w432:dbl)
        n141 = call "LED_Load Current Limit.vi"("Set LED Current Limit?"=w424, "Load Current Limit Range"=w431, "LED Current (Io)"=w429, "DUT Current Limit in"=w412) -> ("Current Limit Range"=w413:dbl, "Current Limit"=w406:dbl)  [unwired: 9 in, 1 out]
        n142 = call <instrlib>:"niDCPower Configure Source Mode With Channels.vi"("error in (no error)"=w433, "source mode"=w448, "channel name"=w408, "instrument handle"=w428) -> ("error out"=w446:errorcluster, "instrument handle out"=w447:refnum<k15>)  [unwired: 6 in]
        n143 = Unbundle By Name(w421) -> ("Max output resistance"=w420:string)
        n144 = call <instrlib>:"niDCPower Configure Output Function.vi"("error in (no error)"=w446, "output function"=w450, "channel name"=w408, "instrument handle"=w447) -> ("error out"=w441:errorcluster, "instrument handle out"=w442:refnum<k15>)  [unwired: 6 out]
        n145 = property class="niDCPower"(reference=w442, error in=w441, "Current Level Autorange"=w440, "Active Channel"=w408, "Source Delay"=0.0 ("Source:Advanced:Source Delay"), "Current Limit Range"=w413, "Current Limit"=w406, "Voltage Level"=0.0 ("Source:DC Voltage:Voltage Level"), "Voltage Level Range"=w414) -> (reference out=w411:refnum<k15>, error out=w410:errorcluster)
        n146 = Fract/Exp String To Number(string=w420) -> (number=w419:dbl)  [unwired: 3 in, 1 out]
        n147 = Delete From Array(array=w427, index=0) -> (deleted portion=w423:dbl, array with subset deleted=w425:dbl[])  [unwired: 1 in]
        n148 = Select(t=w419, s=w424, f=w423) -> (s? t:f=w422:dbl)
        n149 = call <instrlib>:"niDCPower Configure Output Resistance.vi"("error in (no error)"=w410, "resistance"=w422, "channel name"=w408, "instrument handle"=w411) -> ("error out"=w407:errorcluster, "instrument handle out"=w409:refnum<k15>)  [unwired: 6 in]
        n150 = call-poly <instrlib>:"niDCPower Configure Trigger With Channels (Poly).vi"("error in (no error)"=w407, "input terminal"=w435, "channel name"=w408, "instrument handle"=w409) -> ("error out"=w443:errorcluster, "instrument handle out"=w453:refnum<k15>)  [unwired: 6 in]
        n151 = property class="niDCPower"(reference=w453, error in=w443, "Measure When"=w449, "Aperture Time"=w432) -> (reference out=w445:refnum<k15>, error out=w444:errorcluster)
        n152 = call-poly <instrlib>:"niDCPower Configure Trigger With Channels (Poly).vi"("error in (no error)"=w444, "input terminal"=w434, "channel name"=w408, "instrument handle"=w445) -> ("error out"=w451:errorcluster, "instrument handle out"=w452:refnum<k15>)  [unwired: 6 in]
        n153 = call <instrlib>:"niDCPower Commit With Channels.vi"("error in (no error)"=w451, "channel name"=w408, "instrument handle"=w452) -> ("error out"=w417:errorcluster, "instrument handle out"=w437:refnum<k15>)  [unwired: 7 in]
        n154 = Bundle By Name(cluster=w438, "Output Resistance-LED"=w425, "Load out"=w437) -> (w436:T3)
        n155 = Enqueue Element(queue=w418, element="StartSourceAndLoad", error in (no error)=w417) -> (error out=w416:errorcluster)  [unwired: 1 in, 2 out]
      }
      frame "PerformMeasurement-LED" {
        # "Record Measurement values in LED Mode"
        n156 = Unbundle By Name(w468) -> ("Source Voltage-out"=w476:dbl[], "Source Current - out"=w474:dbl[], "Source out"=w480:refnum<k15>, "Source channel name"=w479:string, "Load out"=w478:refnum<k15>, "Load channel name"=w477:string, "Load Voltage-out"=w472:dbl[], "Load Current - out"=w469:dbl[], "LED Mode Completed?"=w457:bool, "Set LED Current Limit?"=w454:bool)
        n157 = call <instrlib>:"niDCPower Fetch Multiple.vi"("instrument handle"=w480, "channel name"=w479, "error in (no error)"=w460) -> ("instrument handle out"=w467:refnum<k15>, "voltage measurements"=w475:dbl[], "current measurements"=w473:dbl[], "error out"=w459:errorcluster)  [unwired: 7 in, 2 out]
        n158 = call <instrlib>:"niDCPower Fetch Multiple.vi"("instrument handle"=w478, "channel name"=w477, "error in (no error)"=w459) -> ("instrument handle out"=w464:refnum<k15>, "voltage measurements"=w471:dbl[], "current measurements"=w470:dbl[], "error out"=w456:errorcluster)  [unwired: 7 in, 2 out]
        n159 = Build Array (concatenate)(w474, w473) -> (w465:dbl[])
        n160 = Build Array (concatenate)(w476, w475) -> (w466:dbl[])
        n161 = Build Array (concatenate)(w469, w470) -> (w462:dbl[])
        n162 = Build Array (concatenate)(w472, w471) -> (w463:dbl[])
        n163 = case shown="False" w457 {
          tunnel: w458 -> [w484 w496]
          tunnel: w456 -> [w482 w495]
          tunnel: [w481 w493] -> w455
          tunnel: w454 -> [w483 _]
          frame False {
            # "LED Mode-Active"
            n164 = case shown="False" w483 {
              tunnel: w484 -> [w487 w491]
              tunnel: w482 -> [w486 w490]
              tunnel: [w485 w489] -> w481
              frame False {
                # "LED Mode- Next Iteration"
                n165 = Enqueue Element(queue=w487, element="ConfigSourcetoSinglePoint-LED", error in (no error)=w486) -> (error out=w485:errorcluster)  [unwired: 1 in, 2 out]
              }
              frame True {
                # "LED Current Limit set - Exit"
                n166 = Enqueue Element(queue=w491, element="Exit", error in (no error)=w490) -> (error out=w489:errorcluster)  [unwired: 1 in, 2 out]
              }
            }
          }
          frame True {
            # "LED Mode Measurement- Completed"
            n167 = Enqueue Element(queue=w496, element="Exit", error in (no error)=w495) -> (error out=w493:errorcluster)  [unwired: 1 in, 2 out]
          }
        }
        n168 = Bundle By Name(cluster=w468, "Source out"=w467, "Source Voltage-out"=w466, "Source Current - out"=w465, "Load out"=w464, "Load Voltage-out"=w463, "Load Current - out"=w462) -> (w461:T3)
      }
      frame "Exit" {
        # "Exit the Measurement"
        n169 = Unbundle By Name(w501) -> ("Source out"=w503:refnum<k15>, "Source channel name"=w506:string, "Load out"=w505:refnum<k15>, "Load channel name"=w504:string)
        n170 = case shown="No Error" w497 {
          selector: w497 -> [w508 w527]
          tunnel: w505 -> [w518 w538]
          tunnel: w504 -> [w519 w533]
          tunnel: w506 -> [w513 w530]
          tunnel: [w514 w526] -> w502
          tunnel: w503 -> [w515 w537]
          tunnel: w501 -> [w511 w529]
          tunnel: [w510 w529] -> w500
          tunnel: w498 -> [w509 w523]
          frame No Error {
            n171 = Release Queue(queue=w509, error in (no error)=w508) -> (error out=w507:errorcluster)  [unwired: 1 in, 2 out]
            n172 = call <instrlib>:"niDCPower Abort With Channels.vi"("error in (no error)"=w507, "channel name"=w519, "instrument handle"=w518) -> ("error out"=w516:errorcluster, "instrument handle out"=w517:refnum<k15>)  [unwired: 7 in]
            n173 = call <instrlib>:"niDCPower Close.vi"("error in (no error)"=w516, "instrument handle"=w517) -> ("error out"=w520:errorcluster)  [unwired: 9 in]
            n174 = call <instrlib>:"niDCPower Abort With Channels.vi"("error in (no error)"=w520, "channel name"=w513, "instrument handle"=w515) -> ("error out"=w522:errorcluster, "instrument handle out"=w521:refnum<k15>)  [unwired: 7 in]
            n175 = Bundle By Name(cluster=w511, "measurement results.Status"="The measurement is performed successfully" ("message")) -> (w510:T3)
            n176 = call <instrlib>:"niDCPower Close.vi"("error in (no error)"=w522, "instrument handle"=w521) -> ("error out"=w514:errorcluster)  [unwired: 9 in]
          }
          frame Error {
            n177 = call <vilib>:"Clear Errors.vi"("error in (no error)"=w527) -> ("error out"=w524:errorcluster)  [unwired: 5 in, 1 out]
            n178 = Release Queue(queue=w523, error in (no error)=w524) -> (error out=w525:errorcluster)  [unwired: 1 in, 2 out]
            n179 = call <instrlib>:"niDCPower Abort With Channels.vi"("error in (no error)"=w525, "channel name"=w533, "instrument handle"=w538) -> ("error out"=w535:errorcluster, "instrument handle out"=w539:refnum<k15>)  [unwired: 7 in]
            n180 = call <instrlib>:"niDCPower Reset With Channels.vi"("error in (no error)"=w535, "channel name"=w533, "instrument handle"=w539) -> ("error out"=w534:errorcluster, "instrument handle out"=w536:refnum<k15>)  [unwired: 7 in]
            n181 = call <instrlib>:"niDCPower Close.vi"("error in (no error)"=w534, "instrument handle"=w536) -> ("error out"=w540:errorcluster)  [unwired: 9 in]
            n182 = call <instrlib>:"niDCPower Abort With Channels.vi"("error in (no error)"=w540, "channel name"=w530, "instrument handle"=w537) -> ("error out"=w542:errorcluster, "instrument handle out"=w541:refnum<k15>)  [unwired: 7 in]
            n183 = call <instrlib>:"niDCPower Reset With Channels.vi"("error in (no error)"=w542, "channel name"=w530, "instrument handle"=w541) -> ("error out"=w531:errorcluster, "instrument handle out"=w532:refnum<k15>)  [unwired: 7 in]
            n184 = call <instrlib>:"niDCPower Close.vi"("error in (no error)"=w531, "instrument handle"=w532) -> ("error out"=w528:errorcluster)  [unwired: 9 in]
            n185 = Merge Errors(w527, w528) -> (w526:errorcluster)
          }
        }
      }
    }
  }
  "error out" <- w22
  "measure call context out" <- w23
  n186 = Unbundle By Name(w8) -> ("Source Voltage-out"=w7:dbl[], "Source Current - out"=w6:dbl[], "Load Voltage-out"=w5:dbl[], "Load Current - out"=w4:dbl[], "measurement results.Status"=w1:string)
  n187 = Bundle By Name(cluster=T1 {"Status"="", "Source voltages"=[0.0], "Load voltages"=[0.0], "Source current"=[0.0], "Load current"=[0.0]} ("measurement results"), "Source voltages"=w7, "Source current"=w6, "Load voltages"=w5, "Load current"=w4, "Status"=w1) -> (→"measurement results":T1)
